vi "initialize.vi"(8 "error in (no error)":errorcluster, 10 "file path (use dialog)":path, 11 "Data Logger in":refnum<class "Data Logger.lvclass">) -> (0 "error out":errorcluster, 3 "Data Logger out":refnum<class "Data Logger.lvclass">)   [LabVIEW 2017, in "Data Logger.lvlib" / "Data Logger.lvclass"]
uses:
  Data Logger.lvclass
  Data Logger.lvclass/Data Logger.ctl
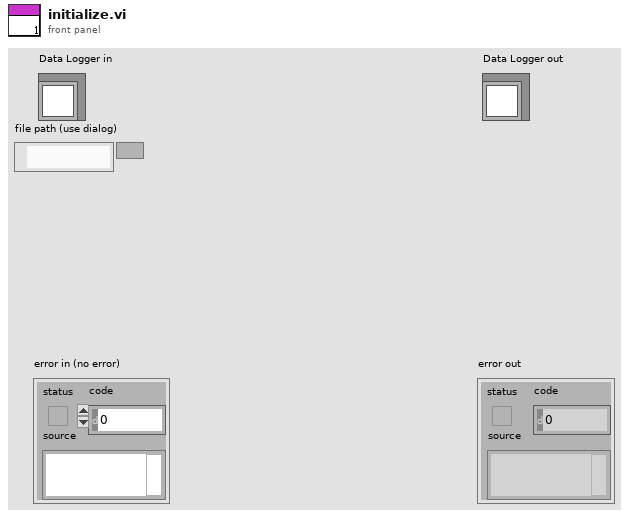
[diagram p1: front panel]
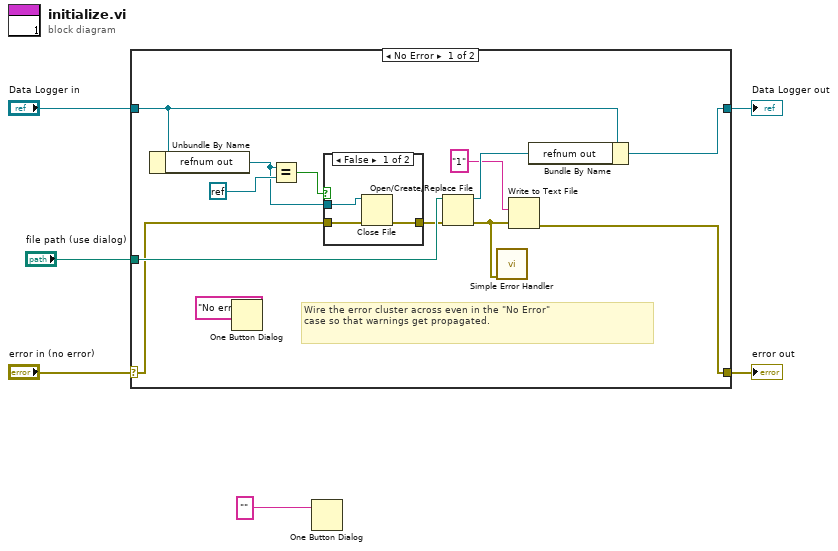
[diagram p0: block diagram]
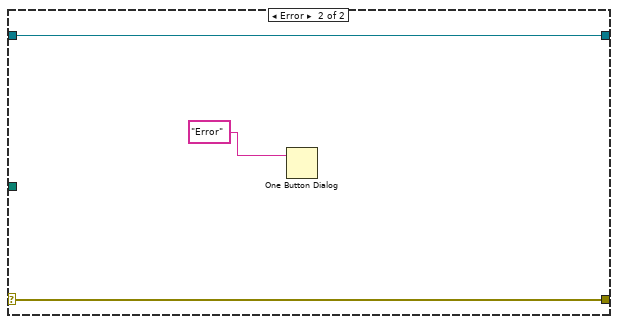
[diagram p3: hidden frame]
diagram:
  n1 = case shown="No Error" "error in (no error)" {
    selector: "error in (no error)" -> [w15 w26]
    tunnel: [w11 w26] -> w5
    tunnel: [w18 w25] -> w3
    tunnel: "Data Logger in" -> [w17 w25]
    tunnel: "file path (use dialog)" -> [w19 _]
    frame No Error {
      # "Wire the error cluster across even in the \"No Error\"\ncase so that warnings get propagated."
      n2 = Unbundle By Name(w17) -> ("refnum out"=w8:refnum<file>)
      n3 = One Button Dialog(message="No error") -> ()  [unwired: 1 in, 1 out]
      n4 = Equal?(x=w8, y=refnum<k0> refnum) -> (x = y?=w9:bool)
      n5 = case shown="False" w9 {
        tunnel: w15 -> [w22 w23]
        tunnel: [w21 w23] -> w14
        tunnel: w8 -> [w20 _]
        frame False {
          n6 = Close File(refnum=w20, error in=w22) -> (error out=w21:errorcluster)  [unwired: 1 out]
        }
        frame True {
        }
      }
      n7 = Open/Create/Replace File(file path (use dialog)=w19, error in=w14) -> (refnum out=w16:refnum<file>, error out=w7:errorcluster)  [unwired: 4 in, 1 out]
      n8 = call <vilib>:"Simple Error Handler.vi"("error in (no error)"=w7) -> ()  [unwired: 4 in, 5 out]
      n9 = Write to Text File(text="1", error in=w7) -> (error out=w11:errorcluster)  [unwired: 2 in, 2 out]
      n10 = Bundle By Name(cluster=w17, "refnum out"=w16) -> (w18:refnum<class "Data Logger.lvclass">)
    }
    frame Error {
      n11 = One Button Dialog(message="Error") -> ()  [unwired: 1 in, 1 out]
    }
  }
  "error out" <- w5
  "Data Logger out" <- w3
  n12 = One Button Dialog(message="") -> ()  [unwired: 1 in, 1 out]
